vi "Unbenannt 4.vi"() -> ()   [LabVIEW 2010]
panel:
  in  "y":fxp<+/-,16,4> format="%.14g"
  out "high?":bool
  out "High":u16
  out "maxhigh2":u16
  in  "Heizen?Mach1":bool
  in  "Mach1maxHigh":u16
  in  "wie viele Messwerte?Mach":u16
  in  "vor der Messung [us]Mach":u16=200
  in  "Per[us]Mach":u16 caption="Abstand zwischen Messungen [us]"
  in  "Abstand zwischen Messungen [us]Mach":u16 caption="Abstand zwischen Messungen [us]"
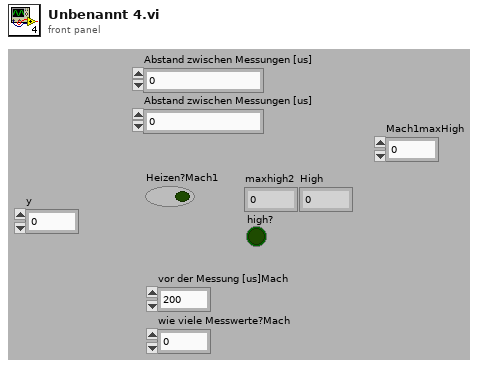
[diagram p1: front panel]
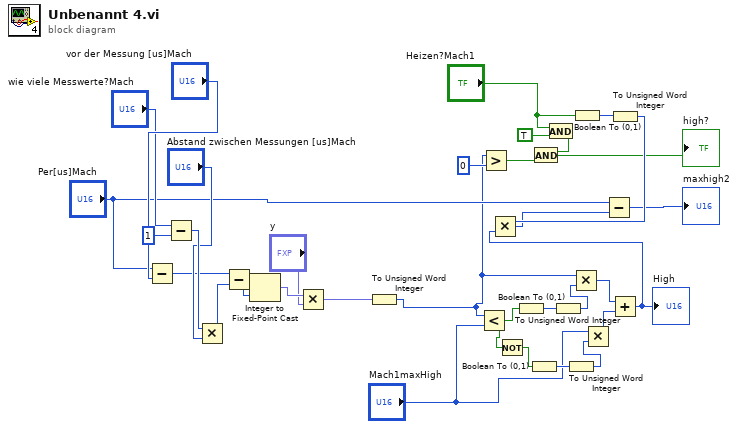
[diagram p0: block diagram]
diagram:
  n1 = Subtract(x="Per[us]Mach", y="vor der Messung [us]Mach") -> (x-y=w28:u16)
  n2 = Subtract(x="wie viele Messwerte?Mach", y=u16 1) -> (x-y=w30:u16)
  n3 = Multiply(x=w30, y="Abstand zwischen Messungen [us]Mach") -> (x*y=w27:u16)
  n4 = Subtract(x=w28, y=w27) -> (x-y=w4:u16)
  n5 = Integer to Fixed-Point Cast ("Integer in Festkomma umwandeln")(integer=w4) -> (fixed-point=w3:fxp<+,16,16>)  [unwired: 1 in]
  n6 = Multiply ("Multiplizieren")(x=w3, y="y") -> (x*y=w1:fxp<+/-,16,16>)
  n7 = To Unsigned Word Integer(number=w1) -> (unsigned 16bit integer=w5:u16)
  n8 = Less?(x=w5, y="Mach1maxHigh") -> (x < y?=w22:bool)
  n9 = Greater?(x=w5, y=u16 0) -> (0:w15:bool)
  n10 = Not(x=w22) -> (.not. x?=w21:bool)
  n11 = Boolean To (0,1)(Boolean=w22) -> (0, 1=w26:i16)
  n12 = Boolean To (0,1)(Boolean=w21) -> (0, 1=w24:i16)
  n13 = And(x="Heizen?Mach1", y=TRUE) -> (x .and. y?=w16:bool)
  n14 = And(x=w16, y=w15) -> (x .and. y?=→"high?":bool)
  n15 = To Unsigned Word Integer(number=w26) -> (unsigned 16bit integer=w25:u16)
  n16 = To Unsigned Word Integer(number=w24) -> (unsigned 16bit integer=w23:u16)
  n17 = Multiply(x=w5, y=w25) -> (x*y=w19:u16)
  n18 = Boolean To (0,1)(Boolean="Heizen?Mach1") -> (0, 1=w13:i16)
  n19 = Multiply(x="Mach1maxHigh", y=w23) -> (x*y=w18:u16)
  n20 = To Unsigned Word Integer(number=w13) -> (unsigned 16bit integer=w12:u16)
  n21 = Add(x=w19, y=w18) -> (x+y=w11:u16)
  "High" <- w11
  n22 = Multiply(x=w12, y=w11) -> (x*y=w10:u16)
  n23 = Subtract(x="Per[us]Mach", y=w10) -> (x-y=→"maxhigh2":u16)
